vi "Error Query.vi"(8 "error in (no error)":errorcluster, 11 "VISA resource name":refnum<visa-resource-name>) -> (0 "error out":errorcluster, 1 "Error Message":string, 2 "Error Code":i32[](array[numeric]), 3 "VISA resource name out":refnum<visa-resource-name>)   [LabVIEW 2023, in "Keysight-DSQx3014T.lvlib"]
doc: "Queries the instrument for any errors in the instrument's error queue. It will continue to read errors until all errors have been read from the instrument. Any errors will be returned in the <B>error out</B> control.\n\n<B>Note(s):</B>\nThis VI is called automatically by most driver VIs so it is not usually necessary to call this in an application."
uses:
  Keysight-DSQx3014T.lvlib
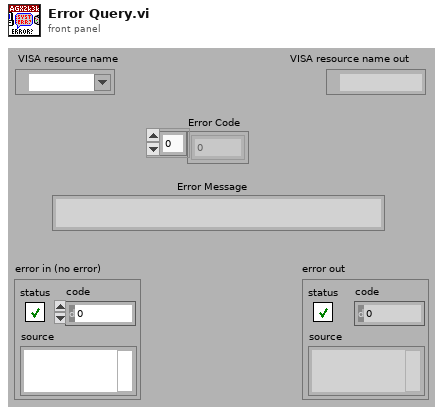
[diagram p1: front panel]
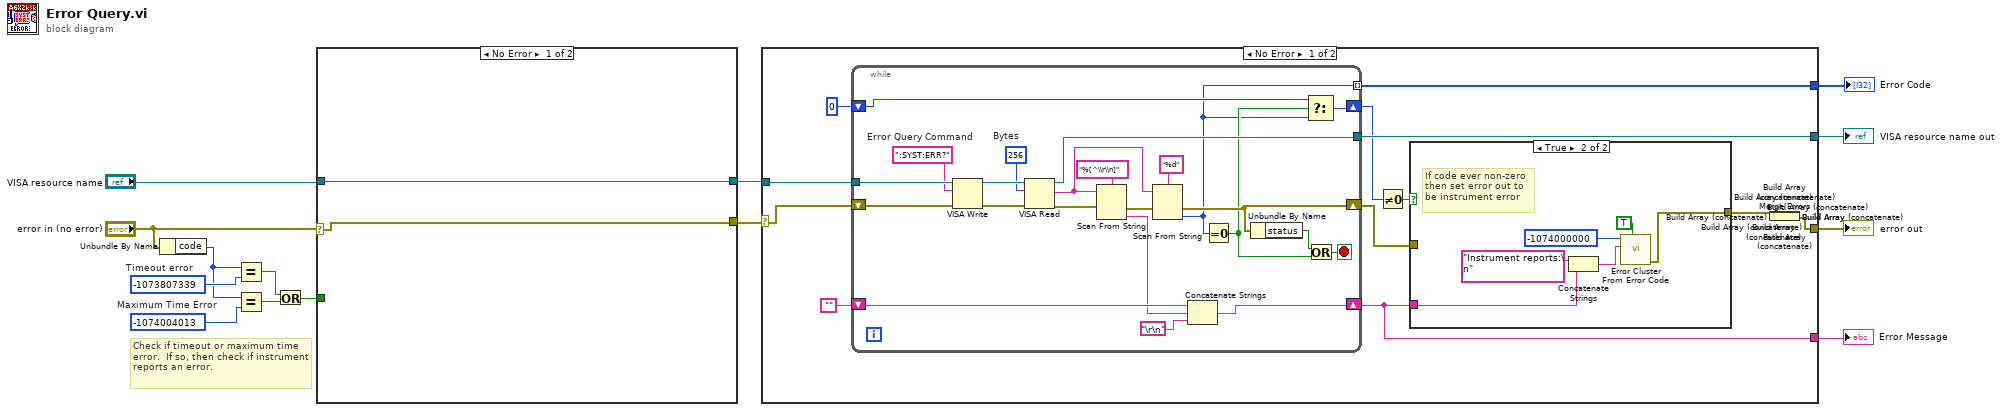
[diagram p0: block diagram]
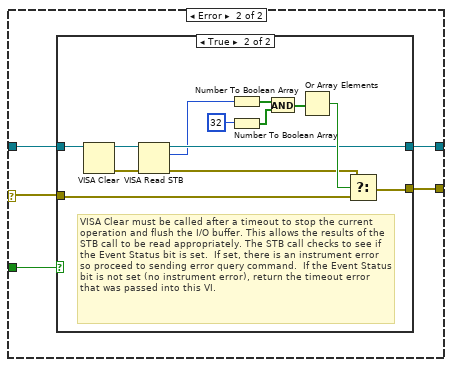
[diagram p2: hidden frame]
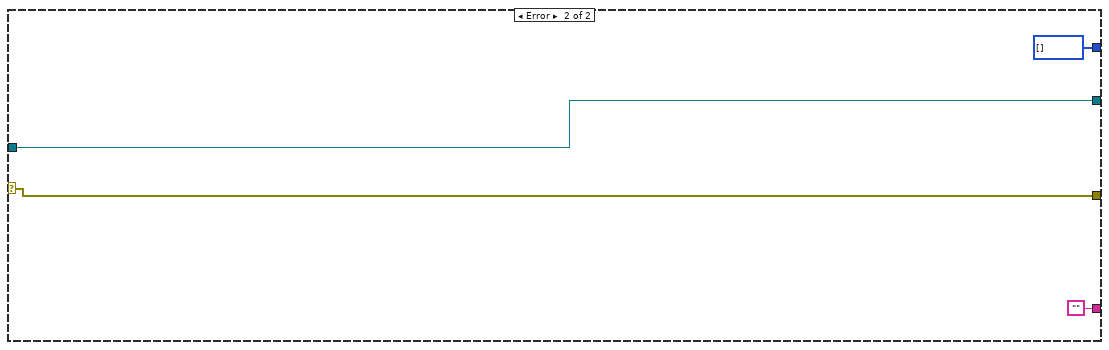
[diagram p5: hidden frame]
diagram:
  w5 = -1074004013  # Maximum Time Error
  w7 = -1073807339  # Timeout error
  # "Check if timeout or maximum time error.  If so, then check if instrument reports an error."
  n1 = Unbundle By Name("error in (no error)") -> ("code"=w6:i32)
  n2 = Equal?(x=w6, y=w7) -> (x = y?=w3:bool)
  n3 = Equal?(x=w6, y=w5) -> (x = y?=w4:bool)
  n4 = Or(x=w3, y=w4) -> (x .or. y?=w2:bool)
  n5 = case shown="No Error" "error in (no error)" {
    selector: "error in (no error)" -> [w15 w19]
    tunnel: "VISA resource name" -> [w16 w21]
    tunnel: [w16 w20] -> w9
    tunnel: [w15 w18] -> w10
    tunnel: w2 -> [_ w17]
    frame No Error {
    }
    frame Error {
      n6 = case shown="True" w17 {
        tunnel: w21 -> [w23 w29]
        tunnel: [w23 w26] -> w20
        tunnel: w19 -> [w22 w32]
        tunnel: [w22 w31] -> w18
        frame False {
          # "Error code not a timeout, so best to pass on to user."
        }
        frame True {
          # "VISA Clear must be called after a timeout to stop the current operation and flush the I/O buffer. This allows the results of the  STB call to be read appropriately. The STB call checks to see if the Event Status bit is set.  If set, there is an instrument error so proceed to sending error query command.  If the Event Status bit is not set (no instrument error), return the timeout error that was passed into this VI."
          n7 = VISA Clear(VISA resource name=w29) -> (VISA resource name out=w28:refnum<visa-resource-name>, error out=w27:errorcluster)  [unwired: 1 in]
          n8 = VISA Read STB(8:w27, 11:w28) -> (0:w25:errorcluster, 2:w24:u16, 3:w26:refnum<visa-resource-name>)
          n9 = Number To Boolean Array(number=w24) -> (Boolean array=w33:bool[])
          n10 = Number To Boolean Array(number=32) -> (Boolean array=w35:bool[])
          n11 = And(x=w33, y=w35) -> (x .and. y?=w34:bool[])
          n12 = Or Array Elements(Boolean array=w34) -> (logical OR=w30:bool)
          n13 = Select(t=w25, s=w30, f=w32) -> (s? t:f=w31:errorcluster)
        }
      }
    }
  }
  n14 = case shown="No Error" w10 {
    selector: w10 -> [w46 w88]
    tunnel: [w57 w91] -> w14
    tunnel: w9 -> [w56 w91]
    tunnel: [w54 w88] -> w13
    tunnel: [w49 ""] -> w12
    tunnel: [w48 i32[] []] -> w11
    frame No Error {
      n15 = while {
        tunnel: [w87] -> w57
        tunnel: w56 -> [w86]
        shift-right: [w74] -> w49
        shift-left: "" -> [w77]
        shift-right: [w72] -> w50
        shift-left: 0 -> [w73]
        shift-right: [w70] -> w47
        shift-left: w46 -> [w71]
        tunnel: [w65] -> w48 mode=indexing
        stop <- w80 stop-if-true
        w84 = u32 256  # Bytes
        w82 = ":SYST:ERR?"  # Error Query Command
        n16 = VISA Write(VISA resource name=w86, write buffer=w82, error in (no error)=w71) -> (VISA resource name out=w85:refnum<visa-resource-name>, error out=w83:errorcluster)  [unwired: 1 out]
        n17 = VISA Read(VISA resource name=w85, byte count=w84, error in (no error)=w83) -> (VISA resource name out=w87:refnum<visa-resource-name>, read buffer=w78:string, error out=w69:errorcluster)  [unwired: 1 out]
        n18 = Scan From String(format string="%[^\\r\\n]", input string=w78, error in=w69) -> (error out=w68:errorcluster, output 1=w75:string)  [unwired: 1 in, 3 out]
        n19 = Scan From String(format string="%d", input string=w78, error in=w68) -> (error out=w70:errorcluster, output 1=w65:i32)  [unwired: 1 in, 3 out]
        n20 = Concatenate Strings(w77, w75, "\r\n") -> (w74:string)
        n21 = Equal To 0?(x=w65) -> (x = 0?=w66:bool)
        n22 = Unbundle By Name(w70) -> ("status"=w67:bool)
        n23 = Select(t=w73, s=w66, f=w65) -> (s? t:f=w72:i32)
        n24 = Or(x=w67, y=w66) -> (x .or. y?=w80:bool)
      }
      n25 = Not Equal To 0?(x=w50) -> (x != 0?=w52:bool)
      n26 = case shown="True" w52 {
        tunnel: w49 -> [_ w63]
        tunnel: [w58 w59] -> w51
        tunnel: w47 -> [w58 _]
        frame False {
        }
        frame True {
          # "If code ever non-zero\nthen set error out to\nbe instrument error"
          n27 = Concatenate Strings("Instrument reports:\n" ("Source"), w63) -> (w60:string)
          n28 = call <vilib>:"Error Cluster From Error Code.vi"("show call chain? (False)"=TRUE, "error message (\"\")"=w60, "error code (0)"=-1074000000 ("Code")) -> ("error out"=w59:errorcluster)  [unwired: 1 in, 5 out]
        }
      }
      n29 = Build Array(w51) -> (w45:errorcluster[])
      n30 = Build Array (concatenate)(w45) -> (w44:errorcluster[])
      n31 = Build Array (concatenate)(w44) -> (w43:errorcluster[])
      n32 = Build Array (concatenate)(w43) -> (w42:errorcluster[])
      n33 = Build Array (concatenate)(w42) -> (w41:errorcluster[])
      n34 = Build Array (concatenate)(w41) -> (w40:errorcluster[])
      n35 = Build Array (concatenate)(w40) -> (w39:errorcluster[])
      n36 = Build Array (concatenate)(w39) -> (w38:errorcluster[])
      n37 = Build Array (concatenate)(w38) -> (w37:errorcluster[])
      n38 = Merge Errors(w37) -> (w54:errorcluster)
    }
    frame Error {
    }
  }
  "VISA resource name out" <- w14
  "error out" <- w13
  "Error Message" <- w12
  "Error Code" <- w11
